vi "6240AData_initialize.vi"(0 "6240AData in":refnum<class "6240AData.lvclass">, 1 "RunIdentifier":string="TEST", 2 "InstName":string="ADCMT", 7 "base path":path=path "C:/LabVIEW/DATA/TestData/Test", 9 "VISA":refnum<visa-resource-name>[](array[refnum])=["GPIB0::1::INSTR", "GPIB0::12::INSTR"], 11 "error in (no error)":errorcluster, 12 "CtrlLabels":string[](array[string])=["6240AX", "6240AY"], 13 "Voltage limits (V)":dbl[](array[numeric])=[12.0, 12.0]) -> (4 "6240AData out":refnum<class "6240AData.lvclass">, 15 "error out":errorcluster={"status"=TRUE, "code"=-1074000000, "source"="ADCMT 6240.lvlib:Error Query.vi<ERR>\nInstrument reports:\n-222,\"Input value is out of the set range\"\r\n0,\"No error\"\r\n\n\n\n<b>Complete call chain:</b>\r\n     ADCMT 6240.lvlib:Error Query.vi\r\n     ADCMT 6240.lvlib:Configure Limiter.vi\r\n     6240AData.lvclass:6240AData_initialize.vi\r\n     Untitled 7"})   [LabVIEW 2017, in "6240AData.lvclass"]
uses:
  6240AData.lvclass
  6240AData.lvclass/6240AData.ctl
  istr.lib/ADCMT 6240/Public/Configure/Configure Output Mode (DC).vi
  istr.lib/ADCMT 6240/ADCMT 6240.lvlib
panel:
  out "Labels":string[](array[string])=["6240AX_state", "6240AX_SetCurrent", "6240AX_ActualVoltage", "6240AX_ActualCurrent", "6240AY_state", "6240AY_SetCurrent", "6240AY_ActualVoltage", "6240AY_ActualCurrent"]
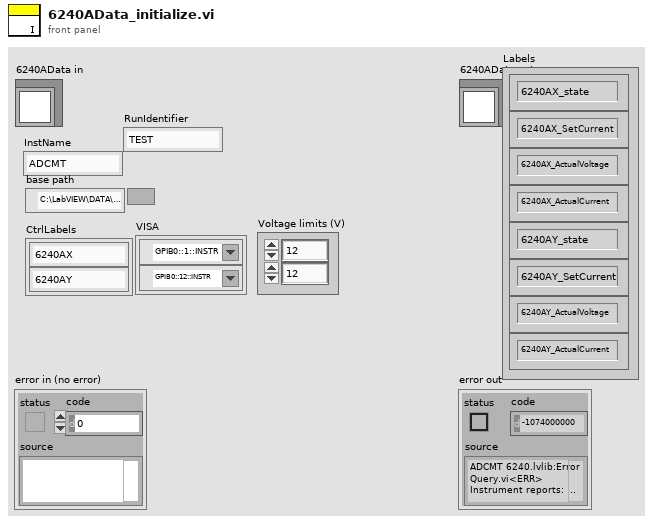
[diagram p1: front panel]
types:
  T1 = enum16{"open", "replace", "create", "open or create", "replace or create", "replace or create with confirmation"}
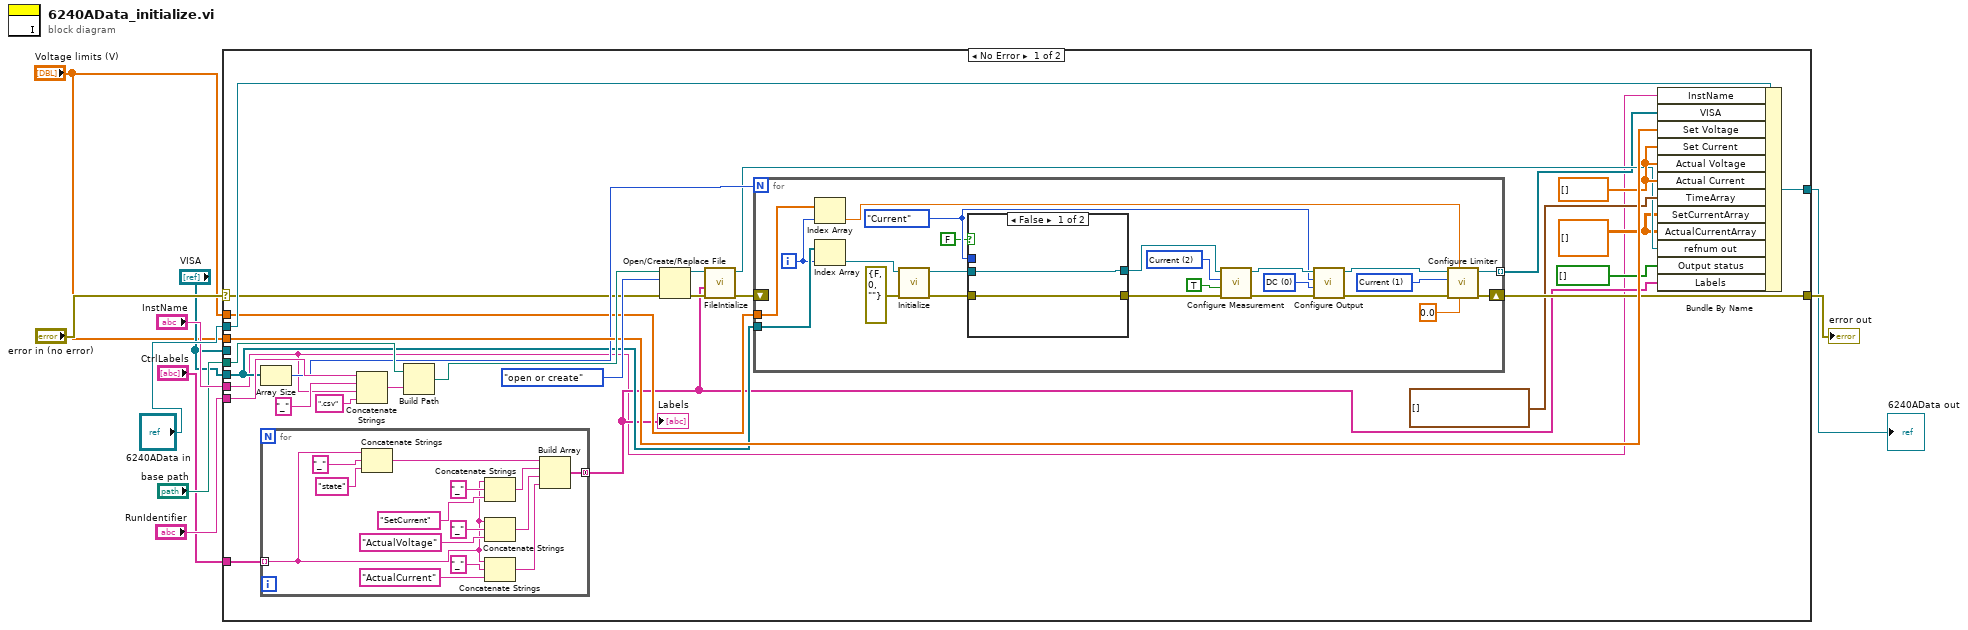
[diagram p0: block diagram]
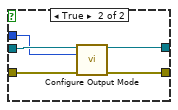
[diagram p2: hidden frame]
diagram:
  n1 = case shown="No Error" "error in (no error)" {
    selector: "error in (no error)" -> [w23 w83]
    tunnel: [w28 w83] -> w9
    tunnel: [w36 w82] -> w7
    tunnel: "6240AData in" -> [w37 w82]
    tunnel: "InstName" -> [w12 _]
    tunnel: "RunIdentifier" -> [w35 _]
    tunnel: "VISA" -> [_ _]
    tunnel: "base path" -> [w33 _]
    tunnel: "Voltage limits (V)" -> [w29 _]
    tunnel: "VISA" -> [w26 _]
    tunnel: "Voltage limits (V)" -> [w25 _]
    tunnel: "CtrlLabels" -> [w21 _]
    frame No Error {
      w15 = dbl[][] [] ("SetCurrentArray")
      w20 = dbl[] [] ("Set Current")
      n2 = Array Size(array=w26) -> (size(s)=w27:i32)
      n3 = for {
        tunnel: w21 -> [w38] mode=indexing
        tunnel: [w42] -> w13 mode=concatenating
        n4 = Concatenate Strings(w38, "_" ("string"), "state" ("string")) -> (w49:string)
        n5 = Concatenate Strings(w38, "_" ("string"), "SetCurrent" ("string")) -> (w50:string)
        n6 = Concatenate Strings(w38, "_" ("string"), "ActualVoltage" ("string")) -> (w51:string)
        n7 = Concatenate Strings(w38, "_" ("string"), "ActualCurrent" ("string")) -> (w39:string)
        n8 = Build Array(w49, w50, w51, w39) -> (w42:string[])
      }
      "Labels" <- w13
      n9 = Concatenate Strings(w35, "_" ("string"), w12, ".csv" ("string")) -> (w32:string)
      n10 = Build Path(base path=w33, name or relative path=w32) -> (appended path=w31:path)
      n11 = Open/Create/Replace File(file path (use dialog)=w31, error in=w23, operation (0:open)=T1."open or create") -> (refnum out=w24:refnum<file>, error out=w22:errorcluster)  [unwired: 3 in, 1 out]
      n12 = call "FileIntialize.vi"("Error In"=w22, "Labels"=w13, "refnum in"=w24) -> ("Error Out"=w17:errorcluster, "File Refnum"=w18:refnum<file>)  [unwired: 7 in]
      n13 = for {
        N: w27 -> [_]
        shift-right: [w61] -> w28
        shift-left: w17 -> [_]
        tunnel: w26 -> [w60]
        tunnel: w25 -> [w58]
        tunnel: [w55] -> w16 mode=indexing
        i -> [w57]
        w54 = u16 1 items=["Voltage", "Current"] ("Source Function  (0: Voltage)")
        w70 = u16 0 items=["DC", "Pulse", "Sweep", "Pulse Sweep", "Pulse-RM"] ("Output Mode  (0: DC)")
        w65 = enum16{"Voltage", "Current"}."Current" ("Source Function  (0: Voltage)")
        w74 = 2 items=["Off", "Volts", "Current", "Resistance"] ("Measurement Function (2: Current)")
        n14 = Index Array(array=w58, index=w57) -> (element=w56:dbl)
        n15 = Index Array(array=w60, index=w57) -> (element=w59:refnum<visa-resource-name>)
        n16 = call "Initialize.vi"("error in (no error)"=errorcluster {"status"=FALSE, "code"=0, "source"=""}, "VISA resource name"=w59) -> ("error out"=w68:errorcluster, "VISA resource name out"=w69:refnum<visa-resource-name>)  [unwired: 8 in]
        n17 = case shown="False" FALSE {
          tunnel: w69 -> [w76 w81]
          tunnel: w68 -> [w75 w80]
          tunnel: [w75 w79] -> w67
          tunnel: [w76 w78] -> w66
          tunnel: w65 -> [_ w77]
          frame False {
          }
          frame True {
            n18 = call-poly "Configure Output Mode.vi"("VISA resource name"=w81, "Source Function  (0: Voltage)"=w77, "error in (no error)"=w80) -> ("VISA resource name out"=w78:refnum<visa-resource-name>, "error out"=w79:errorcluster)  [unwired: 11 in]
          }
        }
        n19 = call "Configure Measurement.vi"("error in (no error)"=w67, "Enable Auto Range (F: Disable)"=TRUE ("Enable Auto Range"), "Measurement Function (2: Current)"=w74, "VISA resource name"=w66) -> ("error out"=w71:errorcluster, "VISA resource name out"=w72:refnum<visa-resource-name>)  [unwired: 6 in]
        n20 = call "Configure Output.vi"("error in (no error)"=w71, "Output Mode  (0: DC)"=w70, "Source Function  (0: Voltage)"=w65, "VISA resource name"=w72) -> ("error out"=w64:errorcluster, "VISA resource name out"=w63:refnum<visa-resource-name>)  [unwired: 6 in]
        n21 = call "Configure Limiter.vi"("Low Limiter Value (-0.3)"=0.0, "Limiter Value (0.3)"=w56, "error in (no error)"=w64, "Source Function  (0: Voltage)"=w54, "VISA resource name"=w63) -> ("error out"=w61:errorcluster, "VISA resource name out"=w55:refnum<visa-resource-name>)  [unwired: 5 in]
      }
      n22 = Bundle By Name(cluster=w37, "InstName"=w12, "VISA"=w16, "Set Voltage"=w29, "Set Current"=w20, "Actual Voltage"=w20, "Actual Current"=w20, "TimeArray"=timestamp[] [], "SetCurrentArray"=w15, "ActualCurrentArray"=w15, "refnum out"=w18, "Output status"=bool[] [], "Labels"=w13) -> (w36:refnum<class "6240AData.lvclass">)
    }
    frame Error {
    }
  }
  "error out" <- w9
  "6240AData out" <- w7
